vi "RunStop.vi"() -> ()   [LabVIEW 2018]
uses:
  lib/Snap7.lvlib
panel:
  out "?":string
  out "RUN/STOP":bool
  in  "RUN":bool=TRUE
  in  "?":bool
  out "Status":string="No Error"
  in  "Slot":i32=2
  in  "Rack":i32
  in  "Address IP":string="192.168.1.12"
  # "STOP"
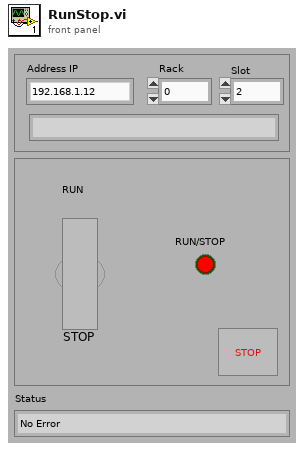
[diagram p1: front panel]
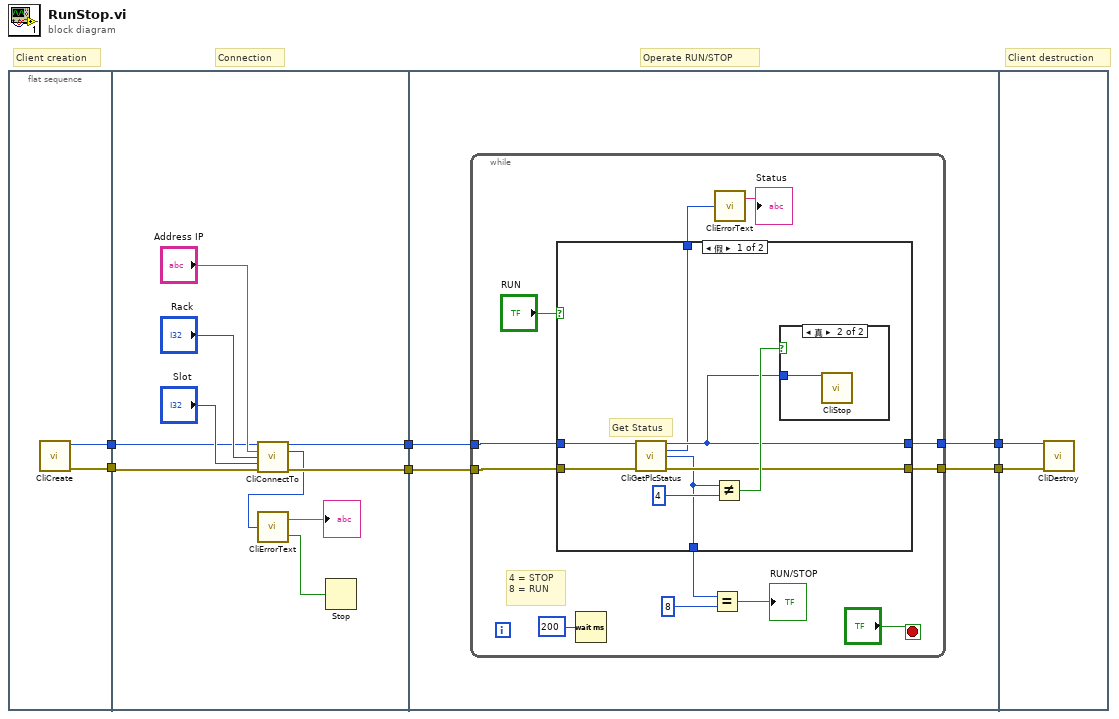
[diagram p0: block diagram]
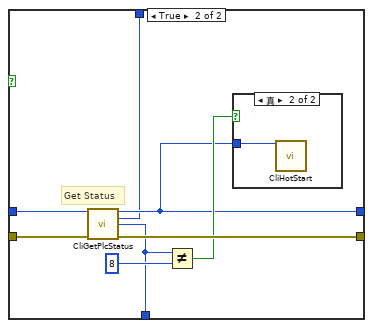
[diagram p3: hidden frame]
diagram:
  # "Client destruction"
  # "Operate RUN/STOP"
  # "Connection"
  # "Client creation"
  n1 = flat-sequence {
    tunnel: [w8] -> w4
    tunnel: [w7] -> w3
    tunnel: [w18] -> w6
    tunnel: [w12] -> w5
    tunnel: w4 -> [w14]
    tunnel: w3 -> [w13]
    tunnel: w6 -> [w22]
    tunnel: w5 -> [w21]
    tunnel: [w20] -> w2
    tunnel: [w19] -> w1
    tunnel: w2 -> [w54]
    tunnel: w1 -> [w53]
    frame #0 {
      n2 = call "CliCreate.vi"() -> ("ref out"=w8:u64, "error out"=w7:errorcluster)  [unwired: 14 in]
    }
    frame #1 {
      n3 = call "CliConnectTo.vi"("ref in"=w14, "Address"="Address IP", "Rack"="Rack", "Slot"="Slot", "error in (no error)"=w13) -> ("ref out"=w12:u64, "Result"=w9:i32, "error out"=w18:errorcluster)  [unwired: 8 in]
      n4 = call "CliErrorText.vi"("ErrNo"=w9) -> ("Error"=w10:bool, "ErrMessage"=→"?":string)
      n5 = Stop(stop? (T)=w10) -> ()
    }
    frame #2 {
      n6 = while {
        tunnel: w21 -> [w30]
        tunnel: w22 -> [w29]
        tunnel: [w28] -> w19
        tunnel: [w27] -> w20
        stop <- "?" stop-if-true
        # "4 = STOP\n8 = RUN"
        n7 = case shown="假" "RUN" {
          tunnel: w30 -> [w40 w51]
          tunnel: w29 -> [w39 w50]
          tunnel: [w37 w48] -> w28
          tunnel: [w38 w46] -> w27
          tunnel: [w36 w45] -> w24
          tunnel: [w35 w44] -> w23
          frame False {
            # "Get Status"
            n8 = call "CliGetPlcStatus.vi"("ref in"=w40, "error in (no error)"=w39) -> ("ref out"=w38:u64, "Result"=w35:i32, "Status"=w36:i32, "error out"=w37:errorcluster)  [unwired: 10 in]
            n9 = Not Equal?(x=w36, y=4 ("x")) -> (x != y?=w41:bool)
            n10 = case shown="真" w41 {
              tunnel: w38 -> [_ w43]
              frame False {
              }
              frame True {
                n11 = call "CliStop.vi"("ref in"=w43) -> ()  [unwired: 12 in, 3 out]
              }
            }
          }
          frame True {
            # "Get Status"
            n12 = call "CliGetPlcStatus.vi"("ref in"=w51, "error in (no error)"=w50) -> ("ref out"=w46:u64, "Result"=w44:i32, "Status"=w45:i32, "error out"=w48:errorcluster)  [unwired: 10 in]
            n13 = Not Equal?(x=w45, y=8 ("x")) -> (x != y?=w47:bool)
            n14 = case shown="真" w47 {
              tunnel: w46 -> [_ w52]
              frame False {
              }
              frame True {
                n15 = call "CliHotStart.vi"("ref in"=w52) -> ()  [unwired: 12 in, 3 out]
              }
            }
          }
        }
        n16 = Wait (ms)(milliseconds to wait=u32 200 ("Loop Delay (ms)")) -> ()  [unwired: 1 out]
        n17 = Equal?(x=w24, y=8) -> (x = y?=→"RUN/STOP":bool)
        n18 = call "CliErrorText.vi"("ErrNo"=w23) -> ("ErrMessage"=→"Status":string)  [unwired: 1 out]
      }
    }
    frame #3 {
      n19 = call "CliDestroy.vi"("ref in"=w54, "error in (no error)"=w53) -> ()  [unwired: 13 in, 1 out]
    }
  }
